vi "Set_Daxsonics.vi"(0 "Daxsonics Settings":T1={"Freq (MHz) "=20, "Voltage (V)"=0, "Gain (dB)"=22} {"Freq (MHz)" items=["4"=4, "6"=6, "8"=8, "10"=10, "12"=12, "15"=15, "17"=17, "20"=20, "25"=25, "30"=30, "35"=35, "40"=40, "45"=45, "50"=50]; "Voltage (V)" items=["0"=0, "10"=10, "20"=20, "30"=30, "40"=40, "50"=50, "60"=60, "70"=70, "80"=80, "90"=90, "100"=100, "110"=110, "120"=120, "130"=130, "140"=140, "150"=150, "160"=160, "170"=170, "180"=180, "190"=190]; "Gain (dB)" items=["22"=22, "25"=25, "28"=28, "31"=31, "34"=34, "37"=37, "40"=40, "43"=43, "46"=46, "49"=49, "52"=52, "55"=55, "58"=58, "61"=61, "64"=64]}, 1 "VISA resource name":refnum<visa-resource-name>="COM8") -> ()   [LabVIEW 2022 SP3]
doc: "This application VI allows the user to set the desired parameters in the \n5800 / 5900 P / R. just select thevalues that you want to set the instrument to from the 5800 / 5900 user interface and click on the send to 5800 button."
uses:
  ScanningControl/Motion Controllers/-MotionRoutines/MotionGlobals.vi
  ScanningControl/Pulsers/Daxsonics/-DaxSubroutines/Dax_Control_Cluster.ctl
panel:
  in  "Freq (MHz)":u16(ring)=1 items=["4", "6", "8", "10", "12", "15", "17", "20", "25", "30", "35", "40", "45", "50"]
  in  "Amp (V)":u16(ring) items=["0", "15", "20", "25", "30", "35", "40", "45", "50", "55", "60", "65", "70", "75", "80", "85", "90", "95", "100"]
  in  "Gain (dB)":u16(ring) items=["0", "3", "6", "9", "12", "15", "18", "21", "24", "27", "30", "33", "36", "39", "42", "45"]
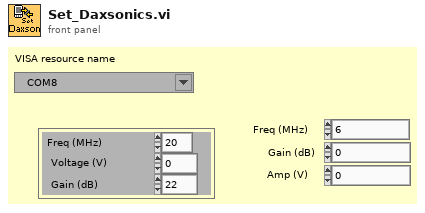
[diagram p1: front panel]
types:
  T1 = typedef "Dax_Control_Cluster.ctl" = cluster{"Freq (MHz) ":u16, "Voltage (V)":u16, "Gain (dB)":u16}
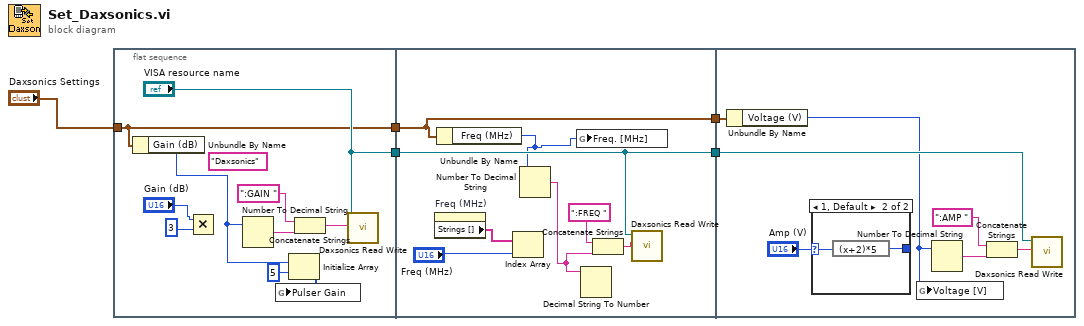
[diagram p0: block diagram]
diagram:
  n1 = flat-sequence {
    tunnel: ["VISA resource name"] -> w5
    tunnel: "Daxsonics Settings" -> [w6]
    tunnel: [w6] -> w3
    tunnel: w5 -> [w19]
    tunnel: [w19] -> w4
    tunnel: w3 -> [w16]
    tunnel: [w16] -> w2
    tunnel: w4 -> [w26]
    tunnel: w2 -> [w25]
    frame #0 {
      (unwired) "Daxsonics" ("string")
      n2 = Unbundle By Name(w6) -> ("Gain (dB)"=w7:u16)
      n3 = Multiply(x="Gain (dB)", y=3) -> ()  [unwired: 1 out]
      n4 = Number To Decimal String(number=w7) -> (decimal integer string=w12:string)  [unwired: 1 in]
      n5 = Initialize Array(w7, 5 ("dimension size")) -> (w9:u16[])
      n6 = global write "MotionGlobals.vi" "Pulser Gain"(w9) -> ()
      n7 = Concatenate Strings(":GAIN " ("string"), w12) -> (w13:string)
      n8 = call "Daxsonics Read Write.vi"("write buffer"=w13, "VISA resource name"="VISA resource name") -> ()  [unwired: 7 in, 3 out]
    }
    frame #1 {
      n9 = property on="Freq (MHz)" class="Ring (strict)"() -> ("Strings []"=w23:string[])  [unwired: 2 in, 2 out]
      n10 = Unbundle By Name(w16) -> ("Freq (MHz)"=w17:u16)
      n11 = Index Array(array=w23, index="Freq (MHz)") -> ()  [unwired: 1 out]
      n12 = Number To Decimal String(number=w17) -> (decimal integer string=w18:string)  [unwired: 1 in]
      n13 = global write "MotionGlobals.vi" "Freq. [MHz]"(w17) -> ()
      n14 = Decimal String To Number(string=w18) -> ()  [unwired: 2 in, 2 out]
      n15 = Concatenate Strings(":FREQ " ("string"), w18) -> (w22:string)
      n16 = call "Daxsonics Read Write.vi"("write buffer"=w22, "VISA resource name"=w19) -> ()  [unwired: 7 in, 3 out]
    }
    frame #2 {
      n17 = Unbundle By Name(w25) -> ("Voltage (V)"=w24:u16)
      n18 = case shown="1, Default" "Amp (V)" {
        selector: "Amp (V)" -> [w31 w33]
        tunnel: [w31 w32] -> _
        frame 0 {
        }
        frame 1, Default {
          n19 = expression code="(x+2)*5"(w33) -> (w32:u16)
        }
      }
      n20 = global write "MotionGlobals.vi" "Voltage [V]"(w24) -> ()
      n21 = Number To Decimal String(number=w24) -> (decimal integer string=w30:string)  [unwired: 1 in]
      n22 = Concatenate Strings(":AMP " ("string"), w30) -> (w29:string)
      n23 = call "Daxsonics Read Write.vi"("write buffer"=w29, "VISA resource name"=w26) -> ()  [unwired: 7 in, 3 out]
    }
  }
